vi "RSI Module_Initialize.vi"(7 "Module Model":T4, 8 "error in (no error)":errorcluster, 9 "Slot Settings":T1, 10 "Channels":T2, 11 "RSI Module in":refnum<class "RSI Module.lvclass">) -> (0 "error out":errorcluster, 3 "RSI Module out":refnum<class "RSI Module.lvclass">)   [LabVIEW 2011, in "Modules.lvlib" / "RSI Module.lvclass"]
uses:
  RSI Module.lvclass
  Module Models.ctl
  Channels.ctl
  Channel Type.ctl
  Slot Settings.ctl
  RSI Module.lvclass/RSI Module.ctl
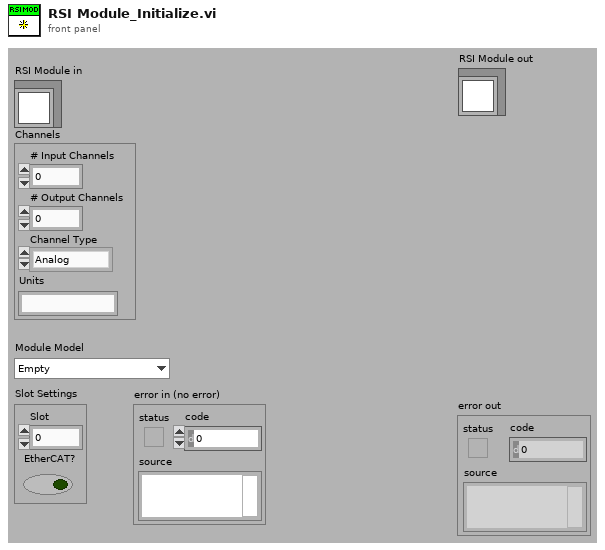
[diagram p1: front panel]
types:
  T1 = typedef "Modules.lvlib/RSI Module.lvclass/Slot Settings.ctl" = cluster{"Slot":u32, "EtherCAT?":bool}
  T2 = typedef "Modules.lvlib/RSI Module.lvclass/Channels.ctl" = cluster{"# Input Channels":i32, "# Output Channels":i32, "Channel Type":T3, "Units":string}
  T3 = typedef "Modules.lvlib/RSI Module.lvclass/Channel Type.ctl" = enum16{"Analog", "Digital"}
  T4 = typedef "Modules.lvlib/RSI Module.lvclass/Module Models.ctl" = enum16{"Empty", "NI 9201", "NI 9203", "NI 9205", "NI 9206", "NI 9207", "NI 9208", "NI 9211", "NI 9213", "NI 9214", "NI 9215", "NI 9217", "NI 9219", "NI 9221", "NI 9225", "NI 9227", "NI 9229", "NI 9233", "NI 9234", "NI 9235", "NI 9236", "NI 9237", "NI 9239", "NI 9263", "NI 9264", "NI 9265", "NI 9269", "NI 9375", "NI 9401", "NI 9402", "NI 9403", "NI 9411", "NI 9421", "NI 9422", "NI 9423", "NI 9425", "NI 9426", "NI 9435", "NI 9472", "NI 9474", "NI 9475", "NI 9476", "NI 9477", "NI 9478", "NI 9481", "NI 9485"}
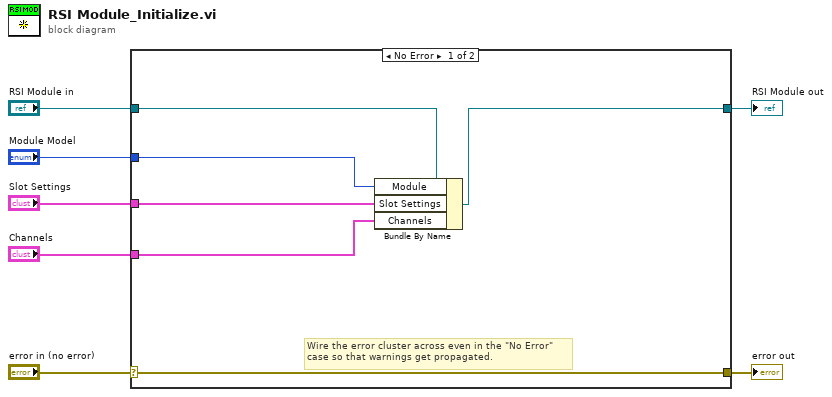
[diagram p0: block diagram]
diagram:
  n1 = case shown="No Error" "error in (no error)" {
    selector: "error in (no error)" -> [w13 w15]
    tunnel: [w13 w15] -> w6
    tunnel: [w12 w14] -> w5
    tunnel: "Module Model" -> [w8 _]
    tunnel: "Channels" -> [w11 _]
    tunnel: "Slot Settings" -> [w9 _]
    tunnel: "RSI Module in" -> [w10 w14]
    frame No Error {
      # "Wire the error cluster across even in the \"No Error\"\ncase so that warnings get propagated."
      n2 = Bundle By Name(cluster=w10, "Module"=w8, "Slot Settings"=w9, "Channels"=w11) -> (w12:refnum<class "RSI Module.lvclass">)
    }
    frame Error {
    }
  }
  "error out" <- w6
  "RSI Module out" <- w5
